vi "Optics_ResetPositionCounter.VI"(8 "Error in":errorcluster, 10 "Motor":dbl, 11 "VISA in":refnum<visa-resource-name>) -> (0 "Error out":errorcluster, 3 "VISA out":refnum<visa-resource-name>)   [LabVIEW 2021]
panel:
  out "String sent":string
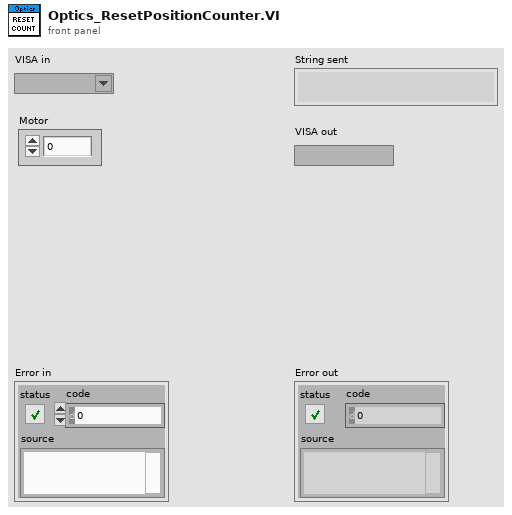
[diagram p1: front panel]
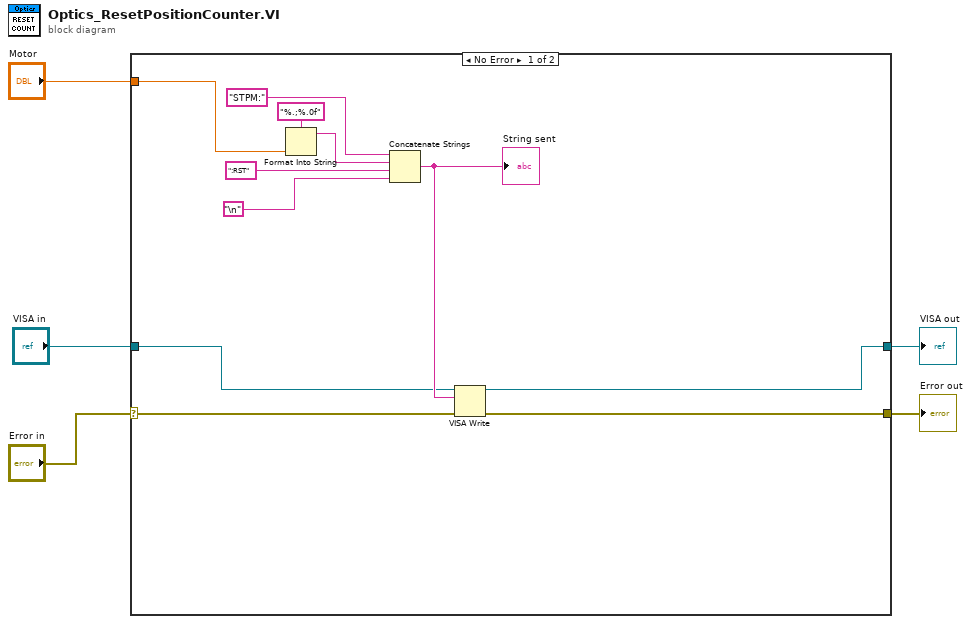
[diagram p0: block diagram]
diagram:
  n1 = case shown="No Error" "Error in" {
    selector: "Error in" -> [w10 w18]
    tunnel: [w9 w18] -> w5
    tunnel: "Motor" -> [w13 _]
    tunnel: "VISA in" -> [w6 w17]
    tunnel: [w8 w17] -> w1
    frame No Error {
      n2 = Format Into String(format string="%.;%.0f", w13) -> (resulting string=w16:string)  [unwired: 2 in, 1 out]
      n3 = Concatenate Strings("STPM:", w16, ":RST", "\n") -> (w11:string)
      "String sent" <- w11
      n4 = VISA Write(VISA resource name=w6, write buffer=w11, error in (no error)=w10) -> (VISA resource name out=w8:refnum<visa-resource-name>, error out=w9:errorcluster)  [unwired: 1 out]
    }
    frame Default {
    }
  }
  "Error out" <- w5
  "VISA out" <- w1
